vi "test udp w fgv.vi"() -> ()   [LabVIEW 2019]
panel:
  out "i":i32
  in  "dt":u32
  in  "data in":string
  in  "정지":bool
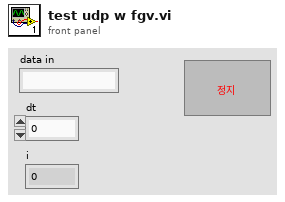
[diagram p1: front panel]
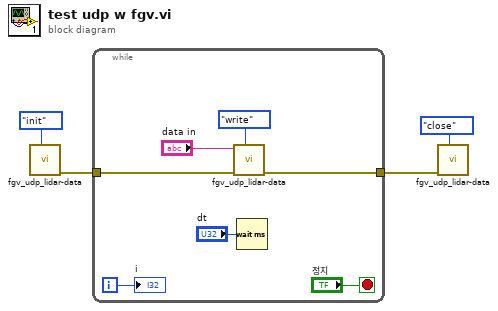
[diagram p0: block diagram]
diagram:
  n1 = call "fgv_udp_lidar-data.vi"("cmd"=enum16{"init", "r-w", "read", "write", "close"}."init") -> ("error out"=w2:errorcluster)  [unwired: 8 in, 2 out]
  n2 = while {
    tunnel: w2 -> [w9]
    tunnel: [w8] -> w1
    i -> [w5]
    stop <- "정지" stop-if-true
    n3 = call "fgv_udp_lidar-data.vi"("cmd"=enum16{"init", "r-w", "read", "write", "close"}."write", "error in"=w9, "data in"="data in") -> ("error out"=w8:errorcluster)  [unwired: 6 in, 2 out]
    n4 = Wait (ms)(milliseconds to wait="dt") -> ()  [unwired: 1 out]
    "i" <- w5
  }
  n5 = call "fgv_udp_lidar-data.vi"("cmd"=enum16{"init", "r-w", "read", "write", "close"}."close", "error in"=w1) -> ()  [unwired: 7 in, 3 out]
